vi "报告打印.vi"(9 "输出簇":T1, 11 "打印?":bool) -> ()   [LabVIEW 2010]
uses:
  <vilib>/Utility/NIReport.llb/NI_report.lvclass
  <vilib>/Utility/NIReport.llb/Append Report Text (str wrap).vi
  全局量/试验配置信息.vi
  <vilib>/addons/_office/word.llb/Word Easy Table (str).vi
  <vilib>/addons/_office/NI_ReportGenerationToolkit.lvlib
  全局量/全局_配置.vi
panel:
  in  "序号":i32
  out "XY图":cluster{"Y":dbl[], "Y":dbl[]}[](graph)
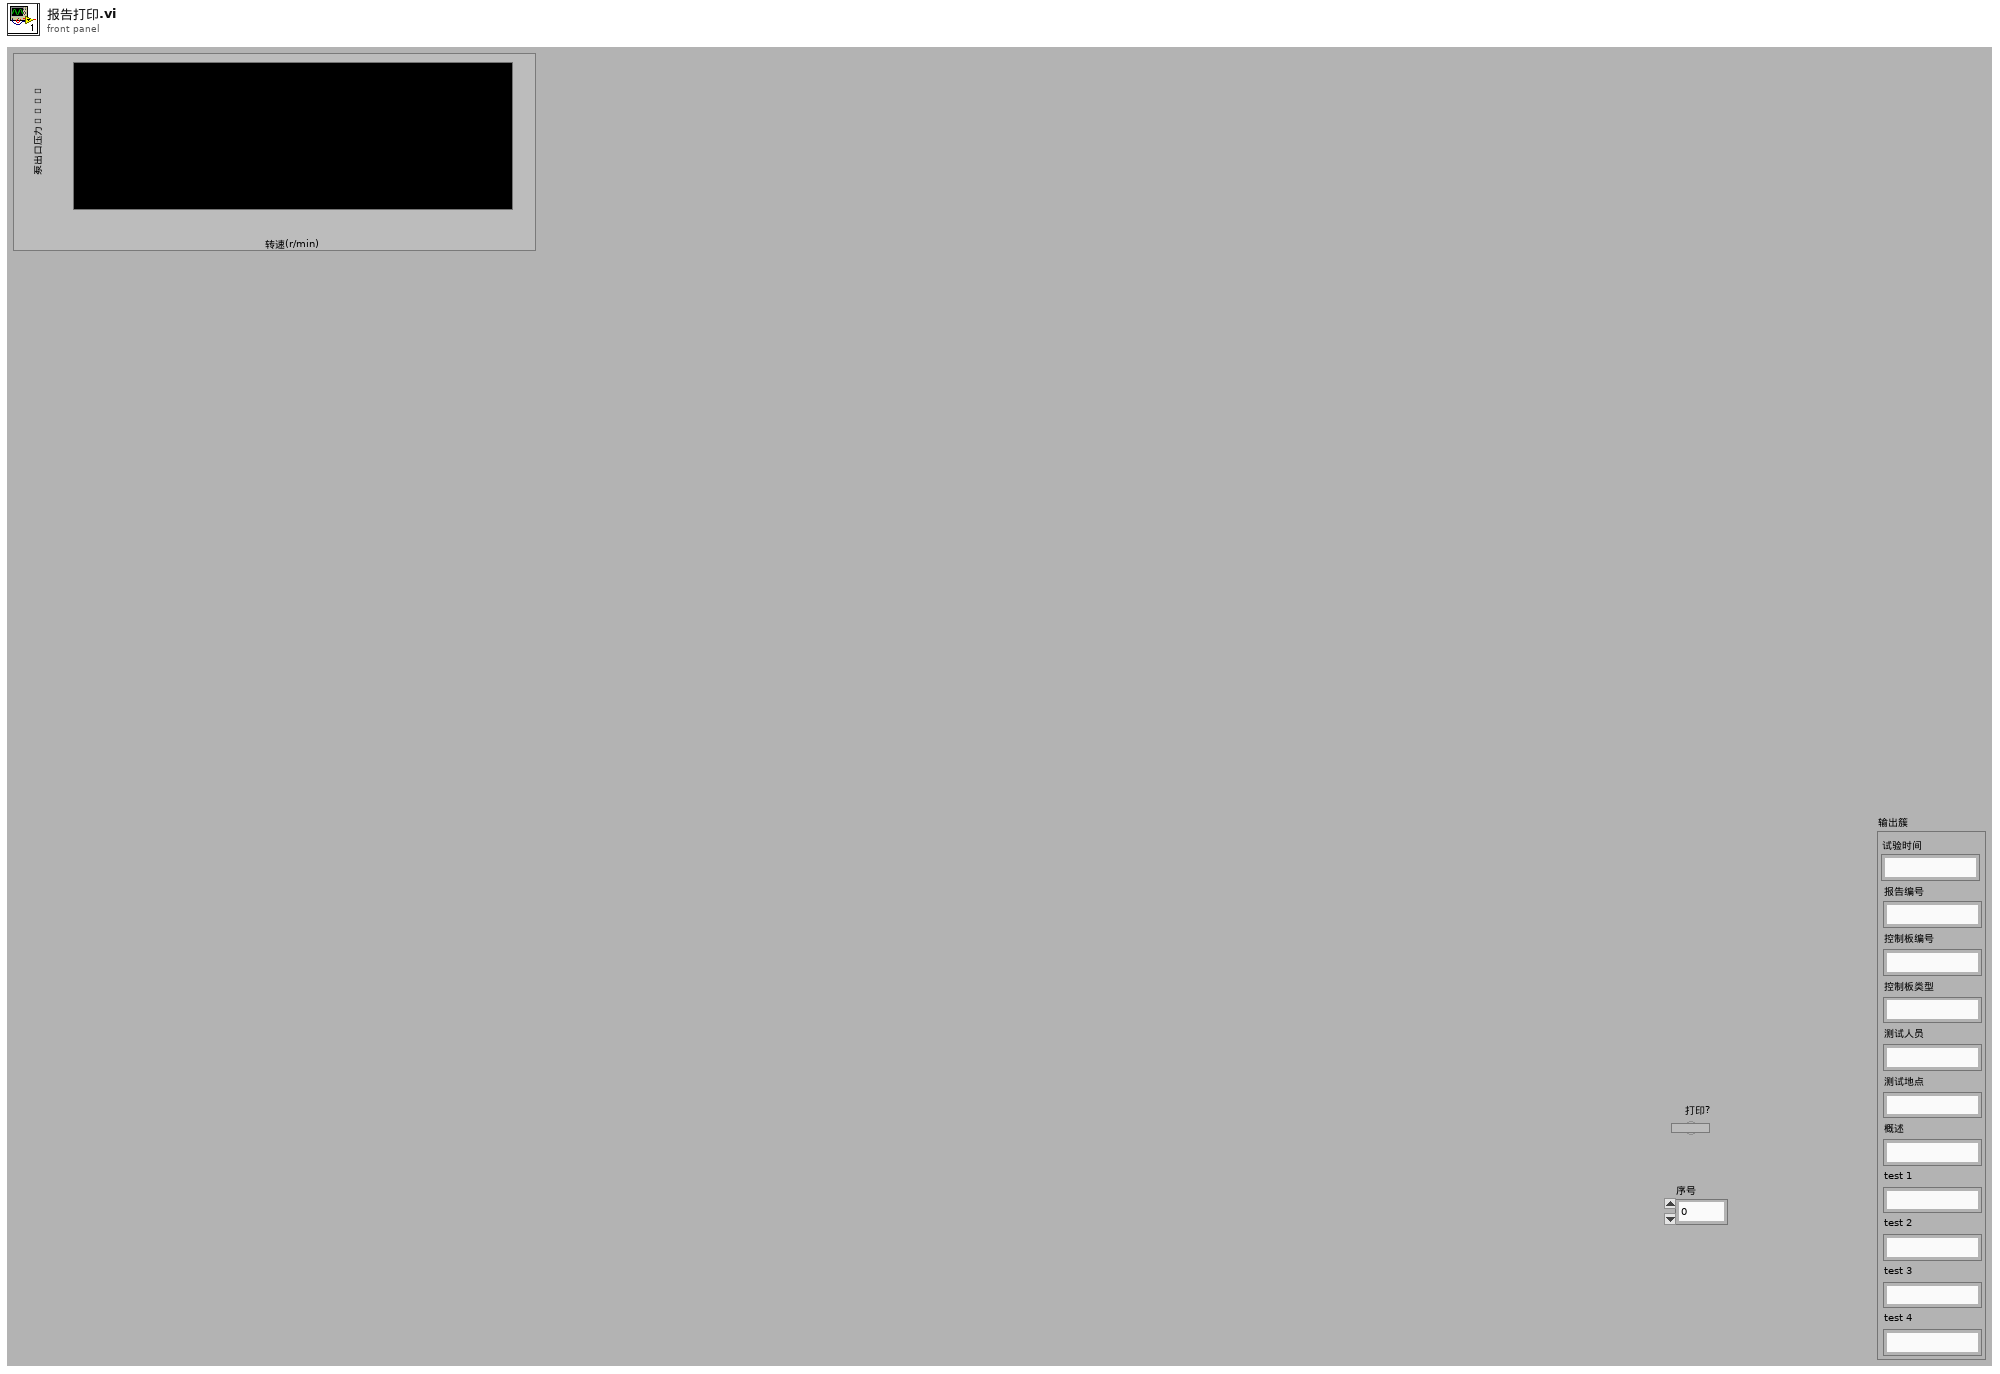
[diagram p1: front panel]
types:
  T1 = cluster{"试验时间":string, "报告编号":string, "控制板编号":string, "控制板类型":string, "测试人员":string, "测试地点":string, "概述":string, "test 1":string, "test 2":string, "test 3":string, "test 4":string}
  T2 = cluster{"position (Excel)":cluster{"row":i32, "column":i32}, "name (Excel)":string, "bookmark (Word)":string}
  T3 = enum16{"maximized", "minimized", "normal", "no change"}
  T4 = enum16{"Standard Report", "HTML", "Word", "Excel"}
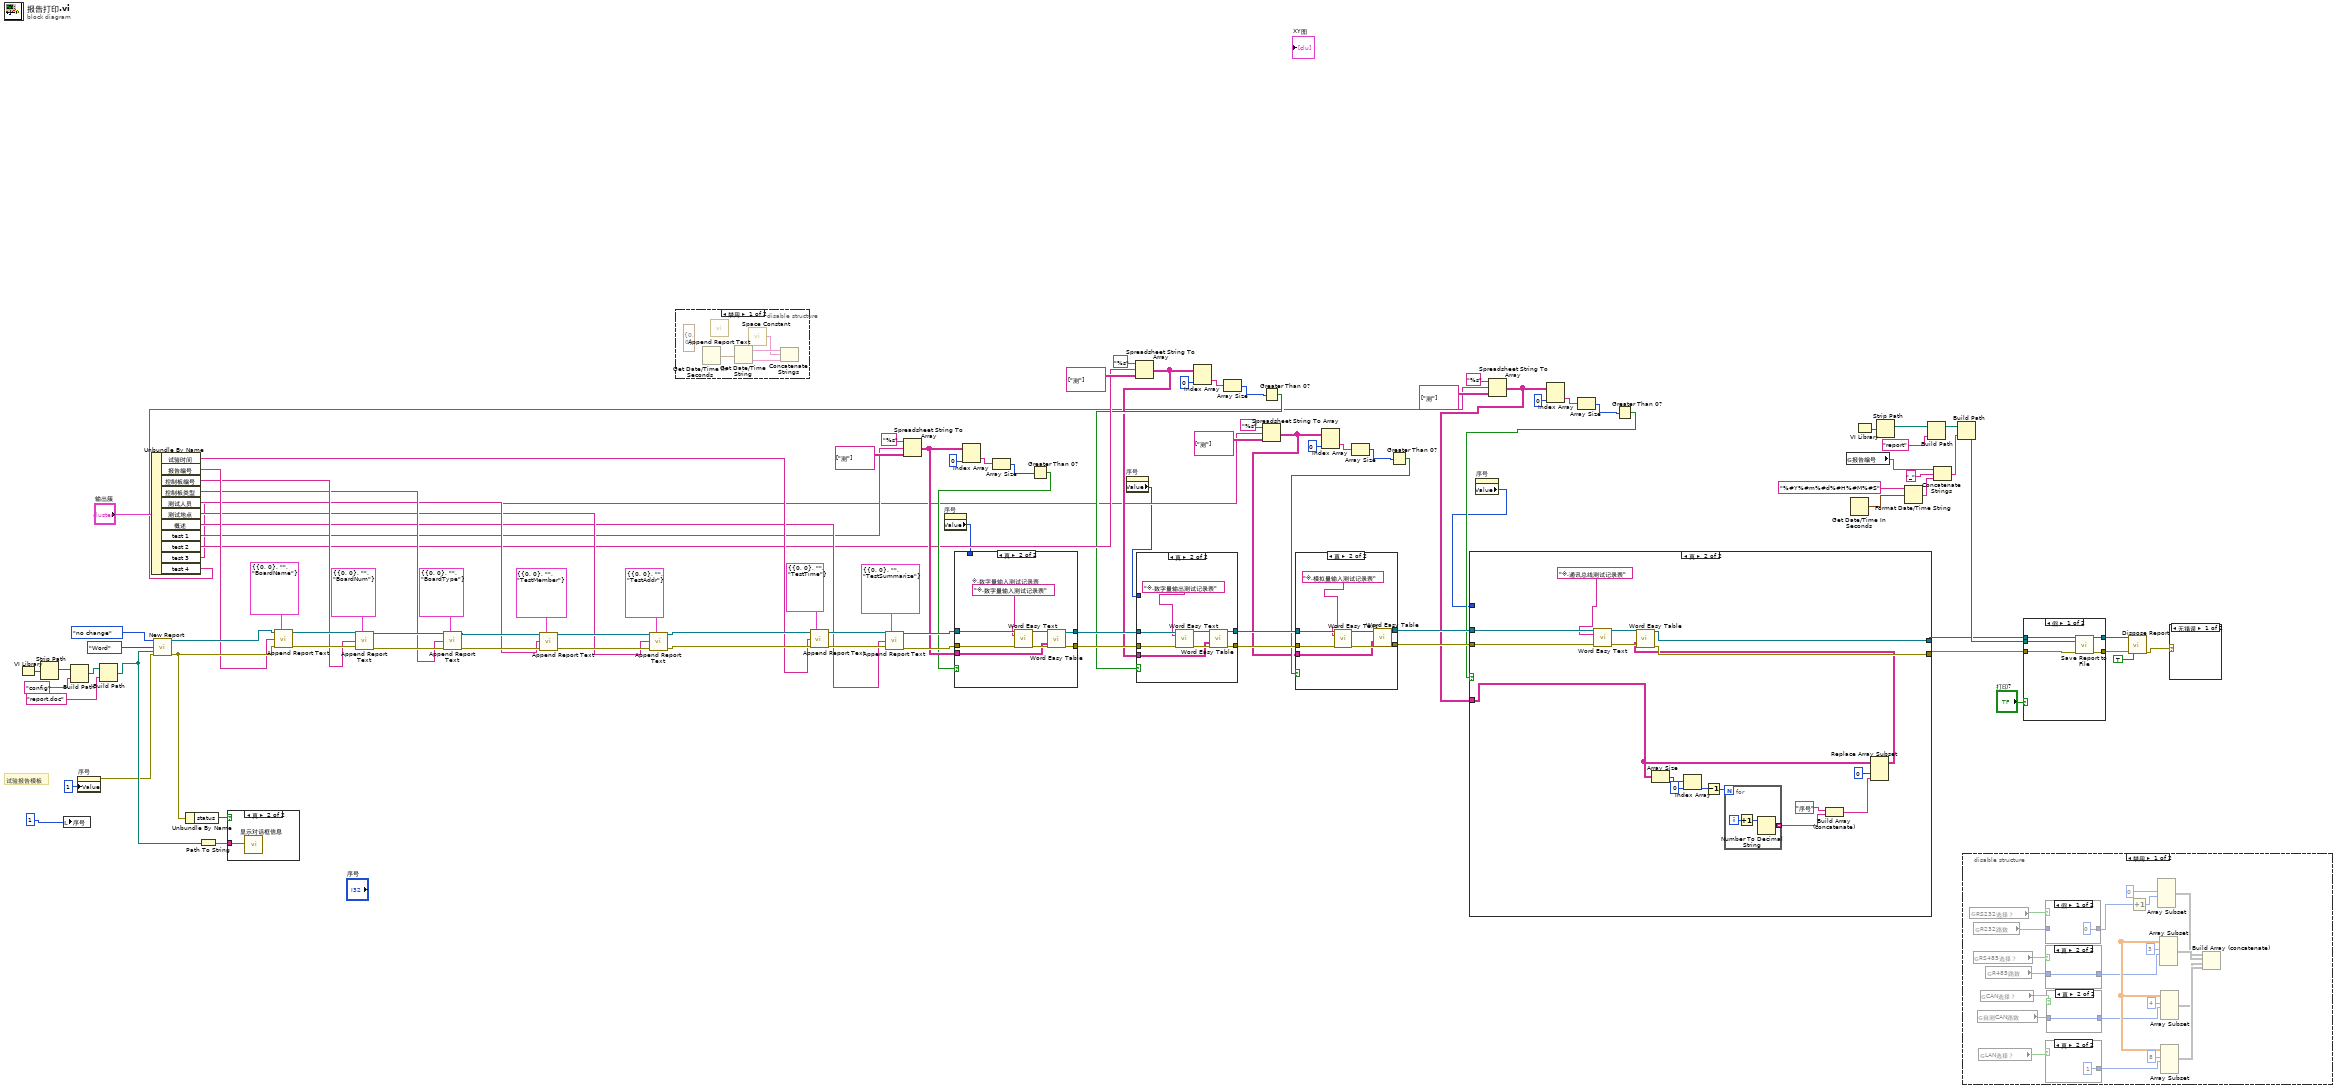
[diagram p0: block diagram]
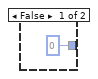
[diagram p2: hidden frame]
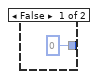
[diagram p3: hidden frame]
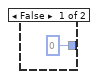
[diagram p5: hidden frame]
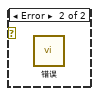
[diagram p11: hidden frame]
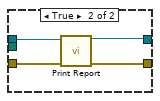
[diagram p12: hidden frame]
diagram:
  # "试验报告模板"
  n1 = VI Library() -> (path=w97:path)
  n2 = Strip Path(path=w97) -> (stripped path=w94:path)  [unwired: 1 out]
  n3 = local write "序号"(1) -> ()
  n4 = Build Path(base path=w94, name or relative path="config") -> (appended path=w96:path)
  n5 = property on="序号" class="DigNum (严格)"("Value"=1 ("序号")) -> (error out=w49:errorcluster)  [unwired: 2 in, 1 out]
  n6 = Build Path(base path=w96, name or relative path="report.doc") -> (appended path=w100:path)
  n7 = Unbundle By Name("输出簇") -> ("试验时间"=w39:string, "报告编号"=w44:string, "控制板编号"=w43:string, "控制板类型"=w42:string, "测试人员"=w41:string, "测试地点"=w40:string, "概述"=w38:string, "test 1"=w35:string, "test 2"=w25:string, "test 3"=w18:string, "test 4"=w11:string)
  n8 = call <vilib>:"New Report.vi"("window state (normal)"=T3."no change", "report type"=T4."Word", "template (empty)"=w100, "error in (no error)"=w49) -> ("report out"=w91:refnum<class "NI_report.lvclass">, "error out"=w90:errorcluster)  [unwired: 10 in]
  n9 = Unbundle By Name(w90) -> ("status"=w102:bool)
  n10 = Path To String(path=w100) -> (string=w101:string)
  n11 = case shown="真" w102 {
    tunnel: w101 -> [_ w104]
    frame False {
    }
    frame True {
      n12 = call "显示对话框信息"("Message"=w104) -> ()  [unwired: 9 in, 2 out]
    }
  }
  n13 = call-poly <vilib>:"Append Report Text.vi"("report in"=w91, "MS Office parameters"=T2 {"position (Excel)"={"row"=0, "column"=0}, "name (Excel)"="", "bookmark (Word)"="BoardName"}, "text"=w44, "error in (no error)"=w90) -> ("report out"=w76:refnum<class "NI_report.lvclass">, "error out"=w75:errorcluster)  [unwired: 8 in, 2 out]
  n14 = call-poly <vilib>:"Append Report Text.vi"("report in"=w76, "MS Office parameters"=T2 {"position (Excel)"={"row"=0, "column"=0}, "name (Excel)"="", "bookmark (Word)"="BoardNum"}, "text"=w43, "error in (no error)"=w75) -> ("report out"=w86:refnum<class "NI_report.lvclass">, "error out"=w85:errorcluster)  [unwired: 8 in, 2 out]
  n15 = call-poly <vilib>:"Append Report Text.vi"("report in"=w86, "MS Office parameters"=T2 {"position (Excel)"={"row"=0, "column"=0}, "name (Excel)"="", "bookmark (Word)"="BoardType"}, "text"=w42, "error in (no error)"=w85) -> ("report out"=w83:refnum<class "NI_report.lvclass">, "error out"=w82:errorcluster)  [unwired: 8 in, 2 out]
  n16 = call-poly <vilib>:"Append Report Text.vi"("report in"=w83, "MS Office parameters"=T2 {"position (Excel)"={"row"=0, "column"=0}, "name (Excel)"="", "bookmark (Word)"="TestMember"}, "text"=w41, "error in (no error)"=w82) -> ("report out"=w80:refnum<class "NI_report.lvclass">, "error out"=w79:errorcluster)  [unwired: 8 in, 2 out]
  n17 = call-poly <vilib>:"Append Report Text.vi"("report in"=w80, "MS Office parameters"=T2 {"position (Excel)"={"row"=0, "column"=0}, "name (Excel)"="", "bookmark (Word)"="TestAddr"}, "text"=w40, "error in (no error)"=w79) -> ("report out"=w78:refnum<class "NI_report.lvclass">, "error out"=w77:errorcluster)  [unwired: 8 in, 2 out]
  n18 = disable-structure shown="禁用" {
    frame Disabled {
      (unwired) cluster{"row":i32, "column":i32} {"row"=0, "column"=0} ("position (excel)")
      n19 = Get Date/Time In Seconds() -> (seconds since 1Jan1904=w108:timestamp)
      n20 = call-poly <vilib>:"Append Report Text.vi"() -> ()  [unwired: 12 in, 4 out]
      n21 = Get Date/Time String(seconds (now)=w108) -> (date string=w107:string, time string=w106:string)  [unwired: 2 in]
      n22 = call <vilib>:"Space Constant.vi"() -> ("String"=w105:string)
      n23 = Concatenate Strings(w107, w105, w106) -> ()  [unwired: 1 out]
    }
    frame Enabled {
    }
  }
  n24 = call-poly <vilib>:"Append Report Text.vi"("report in"=w78, "MS Office parameters"=T2 {"position (Excel)"={"row"=0, "column"=0}, "name (Excel)"="", "bookmark (Word)"="TestTime"}, "text"=w39, "error in (no error)"=w77) -> ("report out"=w54:refnum<class "NI_report.lvclass">, "error out"=w53:errorcluster)  [unwired: 8 in, 2 out]
  n25 = call-poly <vilib>:"Append Report Text.vi"("report in"=w54, "MS Office parameters"=T2 {"position (Excel)"={"row"=0, "column"=0}, "name (Excel)"="", "bookmark (Word)"="TestSummarize"}, "text"=w38, "error in (no error)"=w53) -> ("report out"=w52:refnum<class "NI_report.lvclass">, "error out"=w51:errorcluster)  [unwired: 8 in, 2 out]
  n26 = Spreadsheet String To Array(format string="%s" ("格式字符串"), spreadsheet string=w35, array type (2D Dbl)=string[][] [["测"]] ("数组类型(2D String)")) -> (array=w34:string[][])  [unwired: 1 in]
  n27 = property on="序号" class="DigNum (严格)"() -> ("Value"=w2:i32)  [unwired: 2 in, 2 out]
  n28 = Index Array(array=w34, index (col)=0 ("禁用的索引 (列)")) -> (element=w32:string[])  [unwired: 1 in]
  n29 = Array Size(array=w32) -> (size(s)=w31:i32)
  n30 = Greater Than 0?(x=w31) -> (x > 0?=w30:bool)
  n31 = case shown="真" w30 {
    tunnel: [w110 w117] -> w61
    tunnel: [w109 w116] -> w59
    tunnel: w52 -> [w110 w114]
    tunnel: w51 -> [w109 w113]
    tunnel: w34 -> [_ w112]
    tunnel: w2 -> [_ _]
    frame False {
    }
    frame True {
      w111 = "※.数字量输入测试记录表"  # ※.数字量输入测试记录表
      n32 = call <vilib>:"Word Easy Text.vi"("report in"=w114, "text"=w111, "error in (no error)"=w113) -> ("report out"=w118:refnum<class "NI_report.lvclass">, "error out"=w115:errorcluster)  [unwired: 10 in, 1 out]
      n33 = call-poly <vilib>:"Word Easy Table.vi"("report in"=w118, "data"=w112, "error in (no error)"=w115) -> ("report out"=w117:refnum<class "NI_report.lvclass">, "error out"=w116:errorcluster)  [unwired: 10 in, 1 out]
    }
  }
  n34 = property on="序号" class="DigNum (严格)"() -> ("Value"=w8:i32)  [unwired: 2 in, 2 out]
  n35 = Spreadsheet String To Array(format string="%s" ("格式字符串"), spreadsheet string=w25, array type (2D Dbl)=string[][] [["测"]] ("数组类型(2D String)")) -> (array=w23:string[][])  [unwired: 1 in]
  n36 = Index Array(array=w23, index (col)=0 ("禁用的索引 (列)")) -> (element=w26:string[])  [unwired: 1 in]
  n37 = Array Size(array=w26) -> (size(s)=w7:i32)
  n38 = Greater Than 0?(x=w7) -> (x > 0?=w24:bool)
  n39 = case shown="真" w24 {
    tunnel: w61 -> [w120 w128]
    tunnel: [w120 w126] -> w60
    tunnel: w59 -> [w119 w125]
    tunnel: [w119 w123] -> w58
    tunnel: w8 -> [_ _]
    tunnel: w23 -> [_ w122]
    frame False {
    }
    frame True {
      n40 = call <vilib>:"Word Easy Text.vi"("report in"=w128, "text"="※.数字量输出测试记录表", "error in (no error)"=w125) -> ("report out"=w127:refnum<class "NI_report.lvclass">, "error out"=w124:errorcluster)  [unwired: 10 in, 1 out]
      n41 = call-poly <vilib>:"Word Easy Table.vi"("report in"=w127, "data"=w122, "error in (no error)"=w124) -> ("report out"=w126:refnum<class "NI_report.lvclass">, "error out"=w123:errorcluster)  [unwired: 10 in, 1 out]
    }
  }
  n42 = Spreadsheet String To Array(format string="%s" ("格式字符串"), spreadsheet string=w18, array type (2D Dbl)=string[][] [["测"]] ("数组类型(2D String)")) -> (array=w16:string[][])  [unwired: 1 in]
  n43 = Index Array(array=w16, index (col)=0 ("禁用的索引 (列)")) -> (element=w19:string[])  [unwired: 1 in]
  n44 = Array Size(array=w19) -> (size(s)=w6:i32)
  n45 = Greater Than 0?(x=w6) -> (x > 0?=w17:bool)
  n46 = case shown="真" w17 {
    tunnel: w60 -> [w130 w138]
    tunnel: w58 -> [w129 w136]
    tunnel: [w130 w134] -> w57
    tunnel: [w129 w133] -> w56
    tunnel: w16 -> [_ w132]
    frame False {
    }
    frame True {
      n47 = call <vilib>:"Word Easy Text.vi"("report in"=w138, "text"="※.模拟量输入测试记录表", "error in (no error)"=w136) -> ("report out"=w137:refnum<class "NI_report.lvclass">, "error out"=w135:errorcluster)  [unwired: 10 in, 1 out]
      n48 = call-poly <vilib>:"Word Easy Table.vi"("report in"=w137, "data"=w132, "error in (no error)"=w135) -> ("report out"=w134:refnum<class "NI_report.lvclass">, "error out"=w133:errorcluster)  [unwired: 10 in, 1 out]
    }
  }
  n49 = property on="序号" class="DigNum (严格)"() -> ("Value"=w5:i32)  [unwired: 2 in, 2 out]
  n50 = Spreadsheet String To Array(format string="%s" ("格式字符串"), spreadsheet string=w11, array type (2D Dbl)=string[][] [["测"]] ("数组类型(2D String)")) -> (array=w9:string[][])  [unwired: 1 in]
  n51 = Index Array(array=w9, index (col)=0 ("禁用的索引 (列)")) -> (element=w12:string[])  [unwired: 1 in]
  n52 = Array Size(array=w12) -> (size(s)=w4:i32)
  n53 = Greater Than 0?(x=w4) -> (x > 0?=w10:bool)
  n54 = case shown="真" w10 {
    tunnel: [w140 w157] -> w63
    tunnel: [w139 w156] -> w62
    tunnel: w57 -> [w140 w155]
    tunnel: w56 -> [w139 w154]
    tunnel: w5 -> [_ _]
    tunnel: w9 -> [_ w146]
    frame False {
    }
    frame True {
      n55 = call <vilib>:"Word Easy Text.vi"("report in"=w155, "text"="※.通讯总线测试记录表", "error in (no error)"=w154) -> ("report out"=w153:refnum<class "NI_report.lvclass">, "error out"=w152:errorcluster)  [unwired: 10 in, 1 out]
      n56 = Array Size(array=w146) -> (size(s)=w150:i32[])
      n57 = Index Array(array=w150, index=0 ("索引")) -> (element=w145:i32)
      n58 = Decrement(x=w145) -> (x-1=w144:i32)
      n59 = for {
        N: w144 -> [_]
        tunnel: [w158] -> w142 mode=indexing
        i -> [w160]
        n60 = Increment(x=w160) -> (x+1=w159:i32)
        n61 = Number To Decimal String(number=w159) -> (decimal integer string=w158:string)  [unwired: 1 in]
      }
      n62 = Build Array (concatenate)("序号", w142) -> (w141:string[])
      n63 = Replace Array Subset(array=w146, new element=w141, index (col)=0 ("索引 (行)")) -> (w147:string[][])  [unwired: 1 in]
      n64 = call-poly <vilib>:"Word Easy Table.vi"("report in"=w153, "data"=w147, "error in (no error)"=w152) -> ("report out"=w157:refnum<class "NI_report.lvclass">, "error out"=w156:errorcluster)  [unwired: 10 in, 1 out]
    }
  }
  n65 = global read "试验配置信息.vi" "报告编号"() -> (w47:string)
  n66 = Get Date/Time In Seconds() -> (seconds since 1Jan1904=w69:timestamp)
  n67 = VI Library() -> (path=w70:path)
  n68 = Strip Path(path=w70) -> (stripped path=w73:path)  [unwired: 1 out]
  n69 = Format Date/Time String(time format string (%c)="%#Y%#m%#d%#H%#M%#S" ("时间格式字符串(%c)"), seconds (now)=w69) -> (date/time string=w48:string)  [unwired: 1 in]
  n70 = Build Path(base path=w73, name or relative path="report") -> (appended path=w71:path)
  n71 = Concatenate Strings(w47, "_", w48) -> (w45:string)
  n72 = Build Path(base path=w71, name or relative path=w45) -> (appended path=w65:path)
  n73 = disable-structure shown="禁用" {
    frame Disabled {
      n74 = global read "试验配置信息.vi" "RS232选择？"() -> (w175:bool)
      n75 = global read "试验配置信息.vi" "RS485选择？"() -> (w172:bool)
      n76 = global read "全局_配置.vi" "R232路数"() -> (w174:u32)
      n77 = global read "试验配置信息.vi" "自测CAN路数"() -> (w169:i32)
      n78 = global read "试验配置信息.vi" "LAN选择？"() -> (w168:bool)
      n79 = global read "试验配置信息.vi" "CAN选择？"() -> (w170:bool)
      n80 = global read "全局_配置.vi" "R485路数"() -> (w171:u32)
      n81 = case shown="假" w175 {
        tunnel: w174 -> [_ w187]
        tunnel: [u32 0 ("R232路数") w187] -> w167
        frame False {
        }
        frame True {
        }
      }
      n82 = case shown="真" w172 {
        tunnel: w171 -> [_ w185]
        tunnel: [u32 0 ("R232路数") w185] -> w165
        frame False {
        }
        frame True {
        }
      }
      n83 = case shown="真" w168 {
        tunnel: [u32 0 ("R232路数") u32 1 ("R232路数")] -> w161
        frame False {
        }
        frame True {
        }
      }
      n84 = case shown="真" w170 {
        tunnel: w169 -> [_ w183]
        tunnel: [u32 0 ("R232路数") w183] -> w163
        frame False {
        }
        frame True {
        }
      }
      n85 = Increment(x=w167) -> (x+1=w173:u32)
      n86 = Array Subset(index (row)=0 ("索引"), length (row)=w173) -> (w178:void[][])  [unwired: 3 in]
      n87 = Array Subset(index (row)=3 ("索引"), length (row)=w165) -> (array=w177:dbl[][], w179:void[][])  [unwired: 2 in]
      n88 = Array Subset(array=w177, index (row)=4 ("索引"), length (row)=w163) -> (w180:void[][])  [unwired: 2 in]
      n89 = Array Subset(array=w177, index (row)=8 ("索引"), length (row)=w161) -> (w181:void[][])  [unwired: 2 in]
      n90 = Build Array (concatenate)(w178, w179, w180, w181) -> ()  [unwired: 1 out]
    }
    frame Enabled {
    }
  }
  n91 = case shown="假" "打印?" {
    tunnel: w63 -> [w194 w198]
    tunnel: w62 -> [w193 w197]
    tunnel: [w192 w196] -> w67
    tunnel: [w191 w195] -> w66
    tunnel: w65 -> [w190 _]
    frame False {
      n92 = call-dynamic "Save Report to File.vi"("report in"=w194, "report file path"=w190, "error in (no error)"=w193) -> ("report out"=w192:refnum<class "NI_report.lvclass">, "error out"=w191:errorcluster)  [unwired: 11 in]
    }
    frame True {
      n93 = call-dynamic "Print Report.vi"("report in"=w198, "error in (no error)"=w197) -> ("report out"=w196:refnum<class "NI_report.lvclass">, "error out"=w195:errorcluster)  [unwired: 12 in]
    }
  }
  n94 = call-dynamic "Dispose Report.vi"("report in"=w67, "error in (no error)"=w66, "close report? (T)"=TRUE) -> ("error out"=w64:errorcluster)  [unwired: 12 in]
  n95 = case shown="无错误" w64 {
    frame No Error {
    }
    frame Error {
      n96 = call "错误"() -> ()  [unwired: 10 in, 2 out]
    }
  }
